vi "Log position.vi"(8 "error in (no error)":errorcluster, 11 "StageSPIM in":refnum<class "StageSPIM.lvclass">) -> (0 "error out":errorcluster, 3 "StageSPIM out":refnum<class "StageSPIM.lvclass">)   [LabVIEW 2012, in "StageSPIM.lvclass"]
uses:
  StageSPIM.lvclass
  StageSPIM.lvclass/StageSPIM.ctl
  <vilib>/Utility/file.llb/Write To Spreadsheet File (string).vi
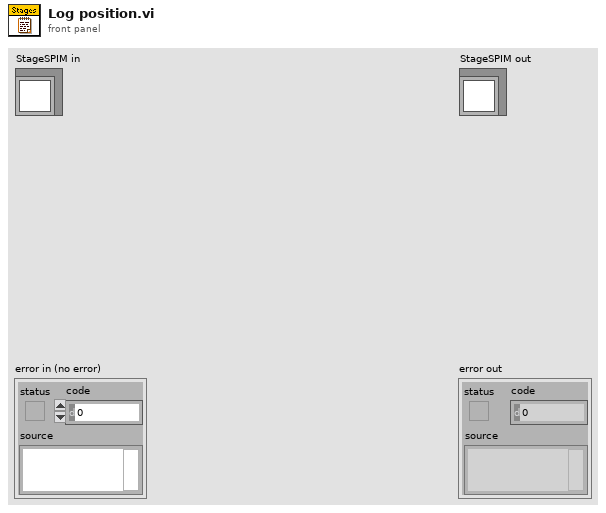
[diagram p1: front panel]
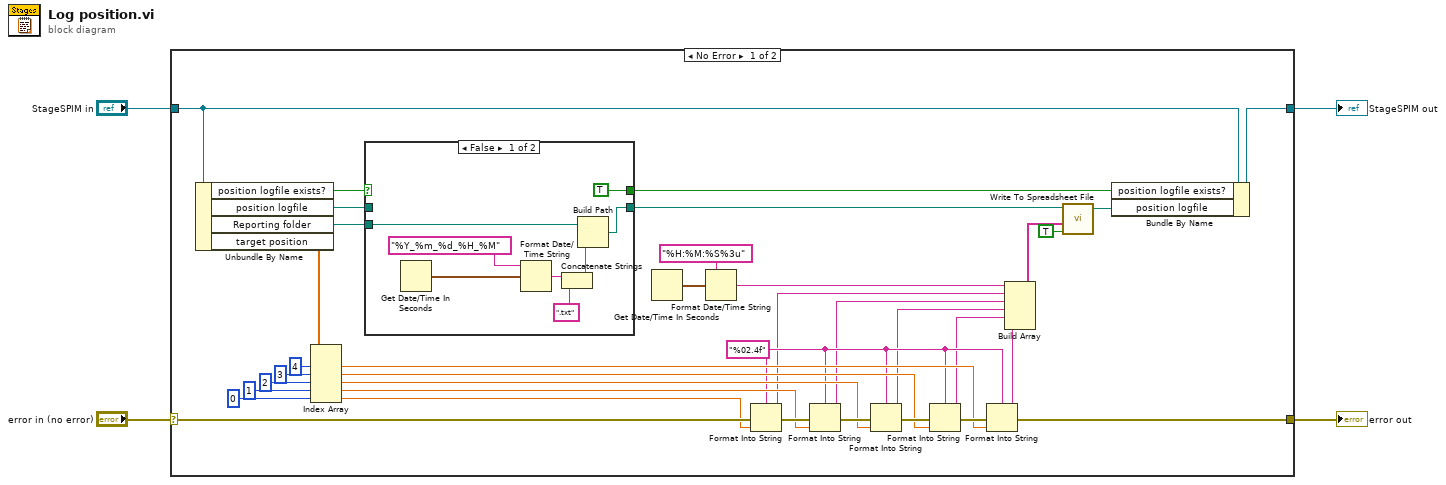
[diagram p0: block diagram]
diagram:
  n1 = case shown="No Error" "error in (no error)" {
    selector: "error in (no error)" -> [w27 w52]
    tunnel: [w26 w52] -> w3
    tunnel: [w7 w51] -> w1
    tunnel: "StageSPIM in" -> [w8 w51]
    frame No Error {
      w20 = "%02.4f" ("format string")
      n2 = Unbundle By Name(w8) -> ("position logfile exists?"=w40:bool, "position logfile"=w38:path, "Reporting folder"=w39:path, "target position"=w37:dbl[])
      n3 = Index Array(array=w37, index #1=4 ("index"), index #2=3 ("index"), index #3=2 ("index"), index #4=1 ("index"), index #5=0 ("index")) -> (element #1=w21:dbl, element #2=w22:dbl, element #3=w23:dbl, element #4=w24:dbl, element #5=w25:dbl)
      n4 = case shown="False" w40 {
        selector: w40 -> [_ w50]
        tunnel: w39 -> [w43 _]
        tunnel: [TRUE w50] -> w5
        tunnel: [w41 w49] -> w10
        tunnel: w38 -> [_ w49]
        frame False {
          n5 = Get Date/Time In Seconds() -> (seconds since 1Jan1904=w45:timestamp)
          n6 = Format Date/Time String(time format string (%c)="%Y_%m_%d_%H_%M", seconds (now)=w45) -> (date/time string=w46:string)  [unwired: 1 in]
          n7 = Concatenate Strings(w46, ".txt" ("string")) -> (w48:string)
          n8 = Build Path(base path=w43, name or relative path=w48) -> (appended path=w41:path)
        }
        frame True {
        }
      }
      n9 = Get Date/Time In Seconds() -> (seconds since 1Jan1904=w19:timestamp)
      n10 = Format Date/Time String(time format string (%c)="%H:%M:%S%3u", seconds (now)=w19) -> (date/time string=w17:string)  [unwired: 1 in]
      n11 = Format Into String(format string=w20, error in=w27, w25) -> (resulting string=w12:string, error out=w31:errorcluster)  [unwired: 1 in]
      n12 = Format Into String(format string=w20, error in=w31, w24) -> (resulting string=w13:string, error out=w30:errorcluster)  [unwired: 1 in]
      n13 = Format Into String(format string=w20, error in=w30, w23) -> (resulting string=w14:string, error out=w29:errorcluster)  [unwired: 1 in]
      n14 = Format Into String(format string=w20, error in=w29, w22) -> (resulting string=w15:string, error out=w28:errorcluster)  [unwired: 1 in]
      n15 = Format Into String(format string=w20, error in=w28, w21) -> (resulting string=w16:string, error out=w26:errorcluster)  [unwired: 1 in]
      n16 = Build Array(w17, w12, w13, w14, w15, w16) -> (w9:string[])
      n17 = call-poly <vilib>:"Write To Spreadsheet File.vi"("append to file? (new file:F)"=TRUE, "1D data"=w9, "file path (dialog if empty)"=w10) -> ("new file path (Not A Path if cancelled)"=w6:path)  [unwired: 5 in]
      n18 = Bundle By Name(cluster=w8, "position logfile exists?"=w5, "position logfile"=w6) -> (w7:refnum<class "StageSPIM.lvclass">)
    }
    frame Error {
    }
  }
  "error out" <- w3
  "StageSPIM out" <- w1
